vi "EventClient_GetEventData.vi"(8 "error in (no error)":errorcluster, 11 "reference":T1) -> (0 "error out":errorcluster, 1 "Data":variant, 3 "reference out":T1)   [LabVIEW 2018]
uses:
  EventClient_ObjectReference.ctl
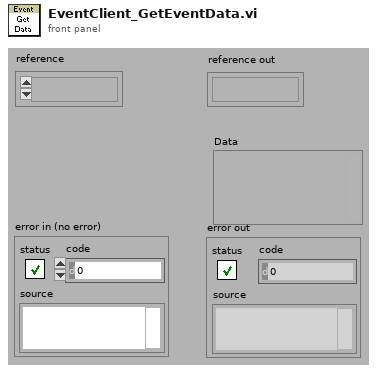
[diagram p1: front panel]
types:
  T1 = typedef "EventClient_ObjectReference.ctl" = refnum<k1>
  T2 = cluster{"Client":refnum<queue>, "Sub Events":string[], "PrvData":variant, "MyName":string}
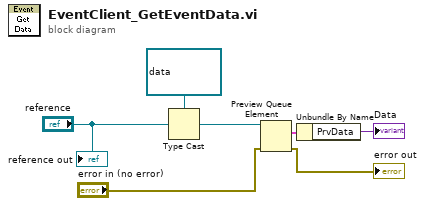
[diagram p0: block diagram]
diagram:
  n1 = Type Cast(type=refnum<queue> refnum ("queue out"), x="reference") -> (*(type *) &x=w6:refnum<queue>)
  n2 = Preview Queue Element(queue=w6, error in (no error)="error in (no error)") -> (element=w5:T2, error out=→"error out":errorcluster)  [unwired: 3 out]
  n3 = Unbundle By Name(w5) -> ("PrvData"=→"Data":variant)
  "reference out" <- "reference"
